vi "Convert ASCII to Alphanumeric Character.vi"(1 "ASCII Value":u8) -> (0 "Alphanumeric Character Value":u16)   [LabVIEW 2015]
panel:
  in  "HT16K33 Alphanumeric LIbrary":u16[](array[numeric])=[1, 2, 4, 8, 16, 32, 64, 128, 256, 512, 1024, 2048, 4096, 8192, 16384, 32768, 0, 0, 0, 0, 0, 0, 0, 0, 4809, 5568, 4857, 227, 1328, 4808, 14848, 5888, 0, 6, 544, 4814, 4845, 3108, 9053, 1024, 9216, 2304, 16320, 4800, 2048, 192, 16384, 3072, 9279, 6, 219, 143, 230, 237, 253, 7, 255, 239, 4608, 2560, 9216, 200, 2304, 4227, 699, 247, 4751, 57, 4623, 249, 113, 189, 246, 4608, 30, 3184, 56, 1334, 8502, 63, 243, 8255, 8435, 237, 4609, 62, 9264, 10294, 11520, 5376, 3081, 57, 8448, 15, 3075, 8, 256, 4184, 8312, 216, 2190, 2136, 113, 1166, 4208, 4096, 14, 13824, 48, 4308, 4176, 220, 368, 1158, 80, 8328, 120, 28, 8196, 10260, 10432, 8204, 2120, 2377, 4608, 9353, 1312, 16383] format=" 0b%016b"
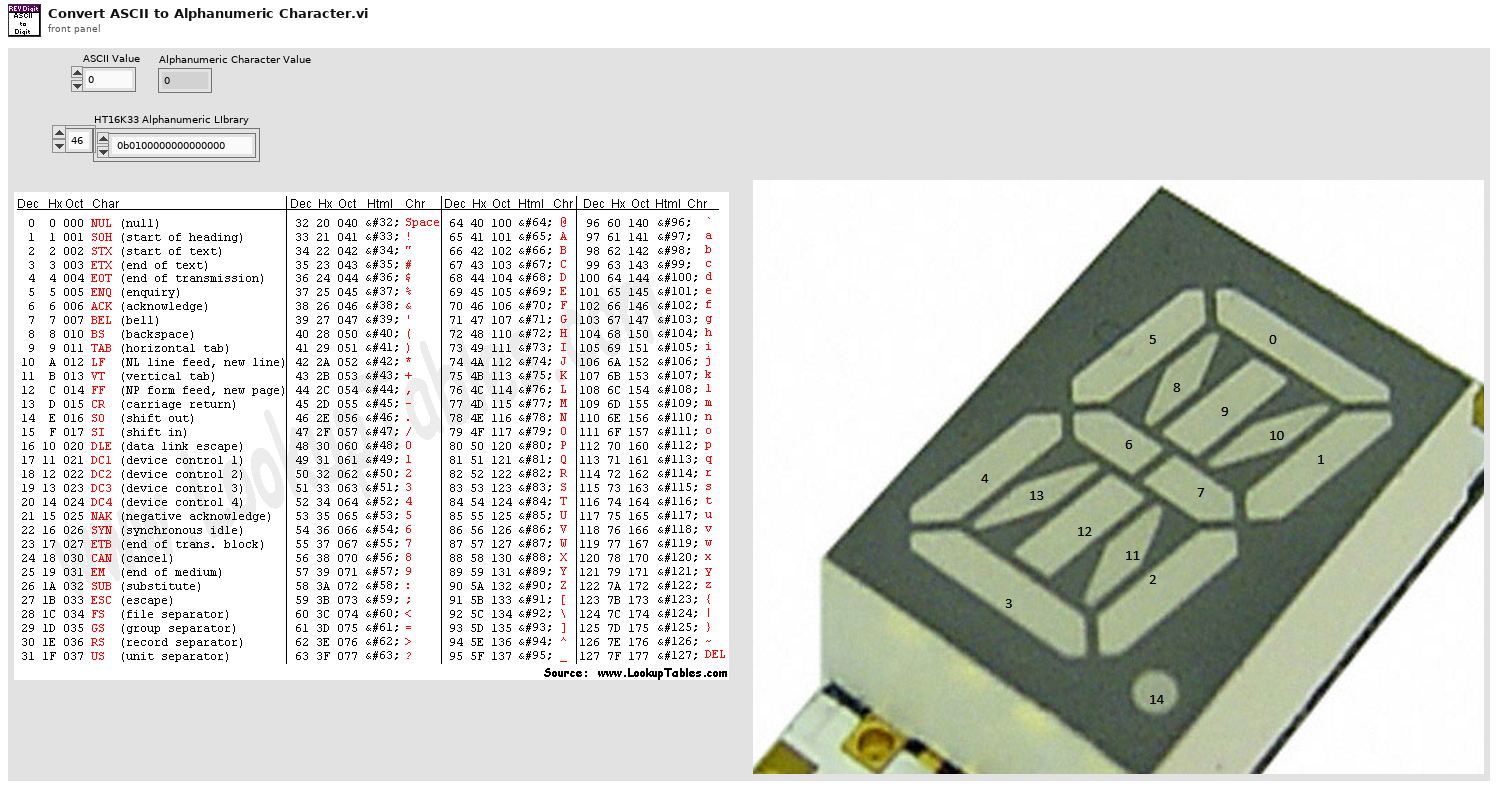
[diagram p1: front panel]
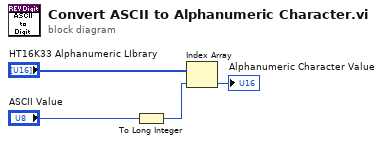
[diagram p0: block diagram]
diagram:
  n1 = To Long Integer(number="ASCII Value") -> (32bit integer=w3:i32)
  n2 = Index Array(array="HT16K33 Alphanumeric LIbrary", index=w3) -> (element=→"Alphanumeric Character Value":u16)
